vi "Check Address Range.vi"(8 "error in (no error)":errorcluster, 10 "Addresses":u32[](array[numeric]) format="%.0x", 11 "Node Pointer In":T1) -> (0 "error out":errorcluster, 2 "Inside NIVS Range":bool[](array[boolean]), 3 "Node Pointer dup":T1)   [LabVIEW 2017, in "GE_RM_System Explorer.lvlib"]
uses:
  GE_RM_System Explorer.lvlib
  <vilib>/NI Veristand/Custom Device API/Custom Device Pointer.ctl
  NationalInstruments.VeriStand.SystemStorage
  <vilib>/NI Veristand/Custom Device API/Custom Device API.lvlib
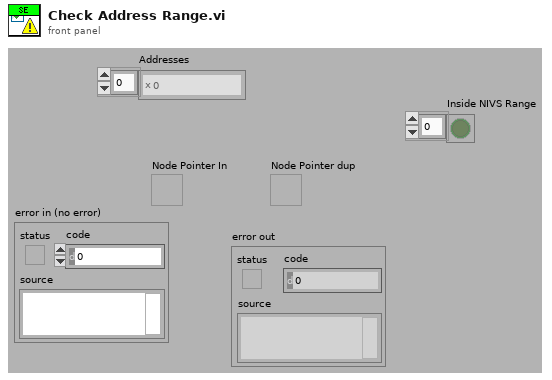
[diagram p1: front panel]
types:
  T1 = typedef "Custom Device API.lvlib/Custom Device Pointer.ctl" = refnum<k24>
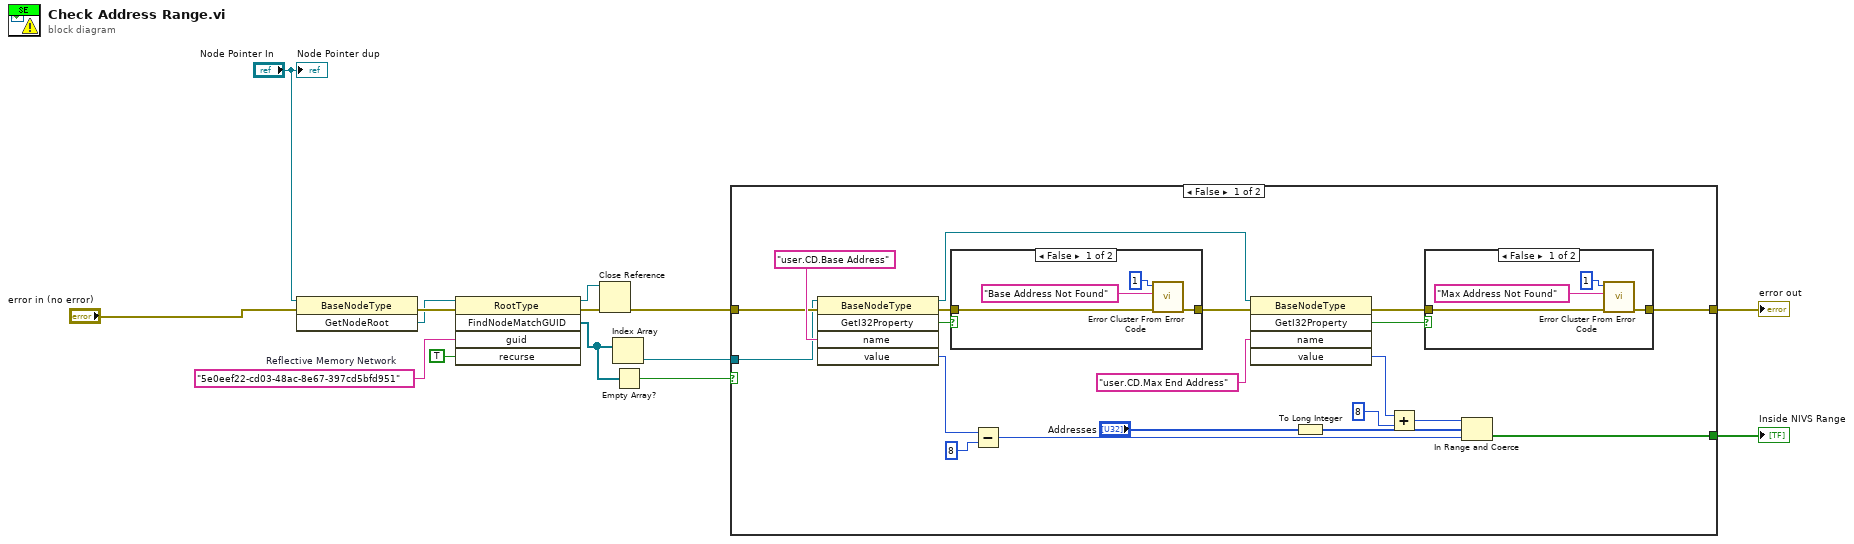
[diagram p0: block diagram]
diagram:
  w5 = "5e0eef22-cd03-48ac-8e67-397cd5bfd951"  # Reflective Memory Network
  n1 = invoke class="BaseNodeType" method="GetNodeRoot"(reference="Node Pointer In", error in="error in (no error)") -> (error out=w8:errorcluster, "GetNodeRoot"=w7:refnum<k24>)  [unwired: 1 in, 1 out]
  n2 = invoke class="RootType" method="FindNodeMatchGUID"(reference=w7, error in=w8, "guid"=w5, "recurse"=TRUE) -> (reference out=w3:refnum<k24>, error out=w4:errorcluster, "FindNodeMatchGUID"=w2:refnum<k24>[])  [unwired: 1 in, 2 out]
  n3 = Close Reference(reference=w3, error in (no error)=w4) -> (error out=w11:errorcluster)
  n4 = Index Array(array=w2) -> (element=w10:refnum<k24>)  [unwired: 1 in]
  n5 = Empty Array?(array=w2) -> (empty?=w9:bool)
  n6 = case shown="False" w9 {
    tunnel: w11 -> [w22 w45]
    tunnel: [w20 w45] -> w12
    tunnel: [w23 _] -> w1
    tunnel: w10 -> [w21 _]
    frame False {
      n7 = invoke class="BaseNodeType" method="GetI32Property"(reference=w21, error in=w22, "name"="user.CD.Base Address") -> (reference out=w33:refnum<k24>, error out=w27:errorcluster, "GetI32Property"=w28:bool, "value"=w30:i32)  [unwired: 2 in, 1 out]
      n8 = case shown="False" w28 {
        tunnel: w27 -> [w43 w44]
        tunnel: [w42 w44] -> w26
        frame False {
          n9 = call <vilib>:"Error Cluster From Error Code.vi"("error in (no error)"=w43, "error message (\"\")"="Base Address Not Found" ("error message (\"\")"), "error code (0)"=1) -> ("error out"=w42:errorcluster)  [unwired: 6 in]
        }
        frame True {
        }
      }
      n10 = Subtract(x=w30, y=8 ("x")) -> (x-y=w18:i32)
      n11 = invoke class="BaseNodeType" method="GetI32Property"(reference=w33, error in=w26, "name"="user.CD.Max End Address") -> (error out=w24:errorcluster, "GetI32Property"=w25:bool, "value"=w31:i32)  [unwired: 2 in, 2 out]
      n12 = To Long Integer(number="Addresses") -> (32bit integer=w29:i32[])
      n13 = Add(x=w31, y=8 ("x")) -> (x+y=w16:i32)
      n14 = case shown="False" w25 {
        tunnel: w24 -> [w38 w39]
        tunnel: [w37 w39] -> w20
        frame False {
          n15 = call <vilib>:"Error Cluster From Error Code.vi"("error in (no error)"=w38, "error message (\"\")"="Max Address Not Found" ("error message (\"\")"), "error code (0)"=1) -> ("error out"=w37:errorcluster)  [unwired: 6 in]
        }
        frame True {
        }
      }
      n16 = In Range and Coerce(upper limit=w16, x=w29, lower limit=w18) -> (In Range?=w23:bool[])  [unwired: 1 out]
    }
    frame True {
    }
  }
  "error out" <- w12
  "Inside NIVS Range" <- w1
  "Node Pointer dup" <- "Node Pointer In"
